vi "PolyCreate.vi"() -> ()   [LabVIEW 2020]
uses:
  <vilib>/Utility/miscctls.llb/LVMapReplaceAction.ctl
  269c9377-1933-43b6-923f-e4fc9fbce505.vi
  <vilib>/Comparison/Equal/Equal Functor/Equal Functor.lvclass
  <vilib>/regexp/Match Regular Expression.xnode
  feature_detection/Apriltag Detector/AprilTag Detector.lvclass
panel:
  out "error out":errorcluster
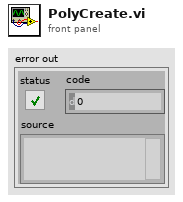
[diagram p1: front panel]
types:
  T1 = typedef "LVMapReplaceAction.ctl" = enum32{"Modify Entry only if found", "Add or Modify Entry", "Delete Entry"}
  T2 = enum32{"invalid VI type", "Standard VI", "Control VI", "Global VI", "Polymorphic VI", "Configuration VI", "SubSystem", "Facade VI", "Method VI", "Statechart Diagram VI"}
  T3 = cluster{"VIPath":path, "Menu Name":string, "Selector Name":string}
  T4 = cluster{"VIPath":path, "Menu Name":string, "Selector Name":string}[]
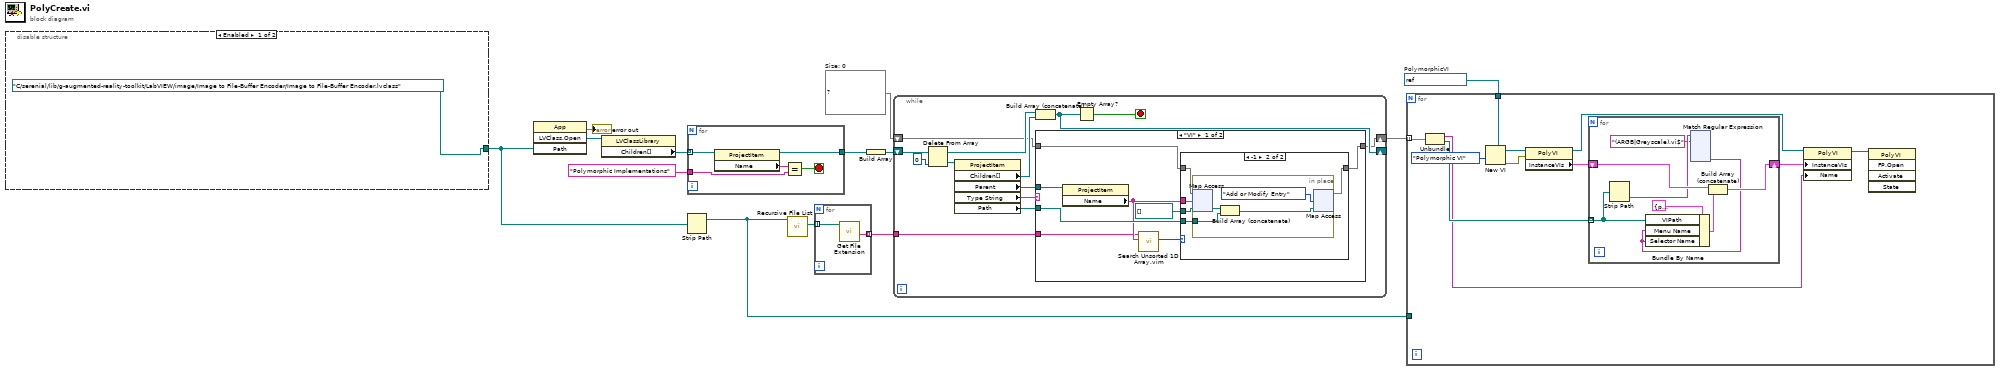
[diagram p0: block diagram]
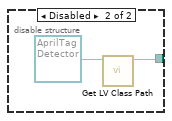
[diagram p2: hidden frame]
diagram:
  w2 = refnum<vi> refnum  # PolymorphicVI
  w8 = map{string, path[]} {}  # Size: 0
  n1 = disable-structure shown="Enabled" {
    disable-tunnel: [path "C:/serenial/lib/g-augmented-reality-toolkit/LabVIEW/image/Image to File-Buffer Encoder/Image to File-Buffer Encoder.lvclass" ("Path") w15] -> w7
    frame Enabled {
    }
    frame Disabled {
      n2 = call <vilib>:"Get LV Class Path.vi"("object"=refnum<class "AprilTag Detector.lvclass"> refnum ("g_ar_toolkit.feature_detection.lvlib:AprilTagDetector.lvclass")) -> ("class path"=w15:path)  [unwired: 9 in, 1 out]
    }
  }
  n3 = invoke class="App" method="LVClass.Open"("Path"=w7) -> (error out=→"error out":errorcluster, "LVClass.Open"=w13:refnum<vi>)  [unwired: 3 in, 2 out]
  n4 = property class="LVClassLibrary"(reference=w13) -> ("Children[]"=w12:refnum<vi>[])  [unwired: 1 in, 2 out]
  n5 = for {
    tunnel: w12 -> [w21] mode=indexing
    tunnel: [w20] -> w11
    tunnel: "Polymorphic Implementations" ("y") -> [w18]
    stop <- w17 stop-if-true
    n6 = property class="ProjectItem"(reference=w21) -> (reference out=w20:refnum<vi>, "Name"=w19:string)  [unwired: 1 in, 1 out]
    n7 = Equal?(x=w19, y=w18) -> (x = y?=w17:bool)
  }
  n8 = Strip Path(path=w7) -> (stripped path=w3:path)  [unwired: 1 out]
  n9 = call <vilib>:"Recursive File List.vi"("Folder Path"=w3) -> ("All Files in Dir"=w6:path[])  [unwired: 6 in, 4 out]
  n10 = for {
    tunnel: w6 -> [w23] mode=indexing
    tunnel: [w22] -> w5 mode=indexing
    n11 = call <vilib>:"Get File Extension.vi"("file"=w23) -> ("filename without extension"=w22:string)  [unwired: 6 in, 4 out]
  }
  n12 = Build Array(w11) -> (w10:refnum<vi>[])
  n13 = while {
    shift-right: [w32] -> _
    shift-left: w10 -> [w36]
    shift-right: [w26] -> w4
    shift-left: w8 -> [w25]
    tunnel: w5 -> [w24]
    stop <- w31 stop-if-true
    n14 = Delete From Array(array=w36, index=0) -> (deleted portion=w34:refnum<vi>, array with subset deleted=w33:refnum<vi>[])  [unwired: 1 in]
    n15 = property class="ProjectItem"(reference=w34) -> ("Children[]"=w29:refnum<vi>[], "Parent"=w28:refnum<vi>, "Type String"=w30:string, "Path"=w27:path)  [unwired: 1 in, 2 out]
    n16 = Build Array (concatenate)(w33, w29) -> (w32:refnum<vi>[])
    n17 = case shown="\"VI\"" w30 {
      tunnel: w28 -> [w44 _]
      tunnel: w27 -> [w42 _]
      tunnel: [w41 w55] -> w26
      tunnel: w25 -> [w40 w55]
      tunnel: w24 -> [w38 _]
      frame "VI" {
        n18 = property class="ProjectItem"(reference=w44) -> ("Name"=w39:string)  [unwired: 1 in, 2 out]
        n19 = call "Search Unsorted 1D Array.vim"("element"=w39, "unsorted 1D array"=w38) -> ("index of element"=w37:i32)  [unwired: 9 in]
        n20 = case shown="-1" w37 {
          tunnel: path[] [] -> [_ w50]
          tunnel: w42 -> [_ w49]
          tunnel: [w45 w48] -> w41
          tunnel: w40 -> [w45 w47]
          tunnel: w39 -> [_ w46]
          frame Default {
          }
          frame -1 {
            n21 = in-place {
              in-place-border: w49 -> [w53]
              n22 = in-place-map #1(w47, w46, w50) -> (w54:path[])  [unwired: 1 out]
              n23 = Build Array (concatenate)(w54, w53) -> (w52:path[])
              n24 = in-place-map #1(w52, LVMapReplaceAction."Add or Modify Entry" ("action")) -> (w48:map{string, path[]})  [unwired: 2 out]
            }
          }
        }
      }
      frame Default {
      }
    }
    n25 = Empty Array?(array=w32) -> (empty?=w31:bool)
  }
  n26 = for {
    tunnel: w4 -> [w66] mode=indexing
    tunnel: w2 -> [w65]
    tunnel: w3 -> [_]
    n27 = Unbundle(w66) -> ("Name"=w58:string, w61:path[])
    n28 = New VI(5:w65, 9:T2."Polymorphic VI" ("vi type (standard vi)")) -> (0:w63:errorcluster, 3:w64:refnum<vi>)  [unwired: 5 in]
    n29 = property class="PolyVI"(reference=w64, error in=w63) -> (reference out=w59:refnum<vi>, "InstanceVIs"=w62:T4)  [unwired: 1 out]
    n30 = for {
      shift-right: [w73] -> w60
      shift-left: w62 -> [w74]
      tunnel: w61 -> [w70] mode=indexing
      n31 = Strip Path(path=w70) -> (name=w69:string)  [unwired: 1 out]
      n32 = xnode "Match Regular Expression"("input string"=w69, "regular expression"="(ARGB|Greyscale).vi$") -> ("submatch 1"=w67:string)  [unwired: 4 in, 5 out]
      n33 = Bundle By Name(cluster=T3 {"VIPath"=path "", "Menu Name"="", "Selector Name"=""}, "VIPath"=w70, "Menu Name"=w67, "Selector Name"=w67) -> (w71:T3)
      n34 = Build Array (concatenate)(w74, w71) -> (w73:T4)
    }
    n35 = property class="PolyVI"(reference=w59, "InstanceVIs"=w60, "Name"=w58) -> (reference out=w57:refnum<vi>)  [unwired: 1 in, 1 out]
    n36 = invoke class="PolyVI" method="FP.Open"(reference=w57) -> ()  [unwired: 4 in, 5 out]
  }
